vi "scene_intersect.vi"(9 "Direction":dbl[](array[numeric]), 10 "Origin":dbl[](array[numeric]), 11 "Spheres":T2[](array[typedef])) -> (0 "N":dbl[](array[numeric]), 1 "Hit":dbl[](array[numeric]), 2 "Material":T1, 3 "SceneIntersect":bool)   [LabVIEW 2015]
uses:
  Sphere.ctl
  Material.ctl
  <vilib>/Analysis/_algsub.llb/Real Vector Norm.vi
  <vilib>/Analysis/NI_AALPro.lvlib
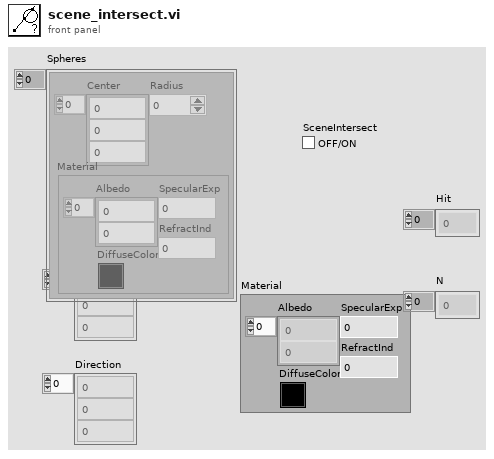
[diagram p1: front panel]
types:
  T1 = typedef "Material.ctl" = cluster{"Albedo":dbl[], "DiffuseColor":u32, "SpecularExp":dbl, "RefractInd":dbl}
  T2 = typedef "Sphere.ctl" = cluster{"Center":dbl[], "Radius":dbl, "Material":T1}
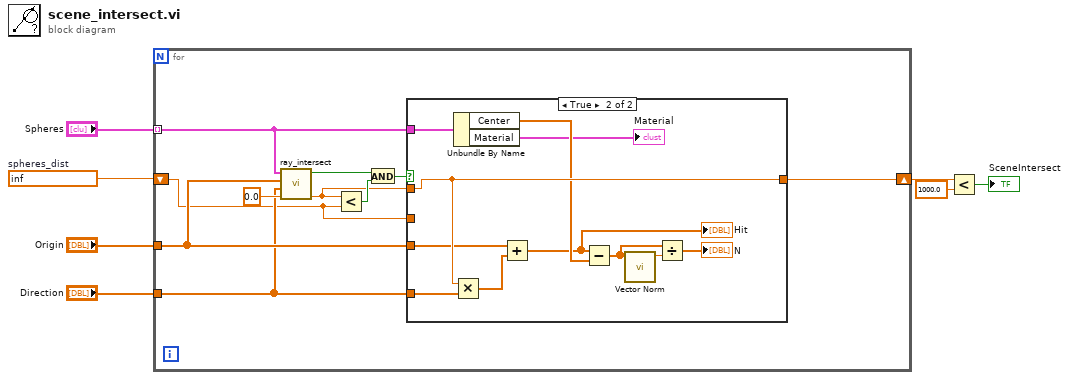
[diagram p0: block diagram]
diagram:
  w4 = inf  # spheres_dist
  n1 = for {
    tunnel: "Spheres" -> [w9] mode=indexing
    tunnel: "Direction" -> [w10]
    tunnel: "Origin" -> [w11]
    shift-right: [w12] -> w3
    shift-left: w4 -> [w8]
    n2 = call "ray_intersect.vi"("Distance"=0.0, "Direction"=w10, "Origin"=w11, "Sphere"=w9) -> ("Distance"=w13:dbl, "RayIntersect"=w16:bool)  [unwired: 6 in]
    n3 = Less?(x=w13, y=w8) -> (x < y?=w15:bool)
    n4 = And(x=w16, y=w15) -> (x .and. y?=w14:bool)
    n5 = case shown="True" w14 {
      tunnel: w13 -> [_ w28]
      tunnel: [w18 w28] -> w12
      tunnel: w11 -> [_ w26]
      tunnel: w10 -> [_ w29]
      tunnel: w9 -> [_ w25]
      tunnel: w8 -> [w18 _]
      frame False {
      }
      frame True {
        n6 = Multiply(x=w28, y=w29) -> (x*y=w27:dbl[])
        n7 = Unbundle By Name(w25) -> ("Center"=w24:dbl[], "Material"=→"Material":T1)
        n8 = Add(x=w26, y=w27) -> (x+y=w20:dbl[])
        "Hit" <- w20
        n9 = Subtract(x=w20, y=w24) -> (x-y=w22:dbl[])
        n10 = call-poly <vilib>:"Vector Norm.vi"("Input Vector"=w22) -> ("norm"=w23:dbl)  [unwired: 9 in, 1 out]
        n11 = Divide(x=w22, y=w23) -> (x/y=→"N":dbl[])
      }
    }
  }
  n12 = Less?(x=w3, y=1000.0) -> (x < y?=→"SceneIntersect":bool)
